vi "ULx Create Channel (AI-Temperature).vi"(0 "task in":refnum<k24>, 5 "physical channels":refnum<k21>, 7 "units":i32(ring) items=["degC", "degF", "kelvin", "raw"], 11 "error in":errorcluster) -> (4 "task out":refnum<k24>, 15 "error out":errorcluster)   [LabVIEW 2020]
doc: "Creates channel(s) to measure temperature."
uses:
  C:/Users/William/Documents/LV 2020 builds/LeaktestDAQ/Source-v33/ULx_LV.dll
  ULx_LV.dll
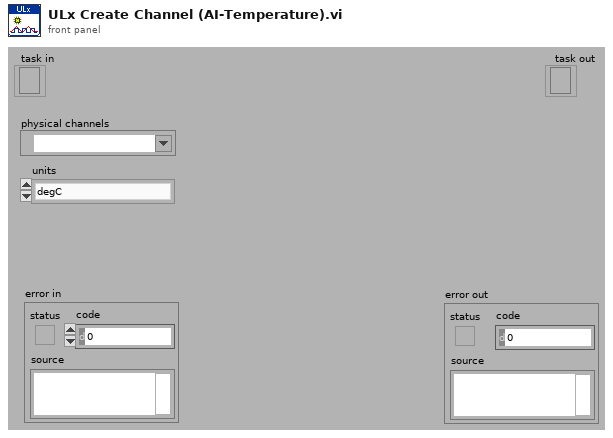
[diagram p1: front panel]
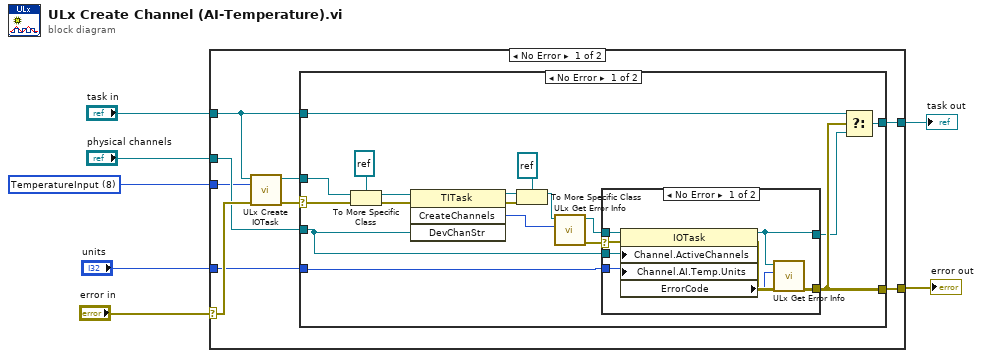
[diagram p0: block diagram]
diagram:
  w2 = 8 items=["AnalogInput", "AnalogOutput", "DigitalInput", "DigitalOutput", "CounterInput", "CounterOutput", "CompositeInput", "CompositeOutput", "TemperatureInput"] ("taskType")
  n1 = case shown="No Error" "error in" {
    selector: "error in" -> [w16 w47]
    tunnel: "task in" -> [w8 w46]
    tunnel: "physical channels" -> [w11 _]
    tunnel: [w14 w46] -> w5
    tunnel: [w13 w47] -> w4
    tunnel: w2 -> [w10 _]
    tunnel: "units" -> [w9 _]
    frame No Error {
      n2 = call "ULx Create IOTask.vi"("error in"=w16, "taskType"=w10, "i/o task in"=w8) -> ("error out"=w15:errorcluster, "i/o task out"=w12:refnum<k24>)  [unwired: 7 in]
      n3 = case shown="No Error" w15 {
        selector: w15 -> [w31 w45]
        tunnel: [w18 w45] -> w13
        tunnel: [w20 w44] -> w14
        tunnel: w12 -> [w29 _]
        tunnel: w11 -> [w25 _]
        tunnel: w9 -> [w26 _]
        tunnel: w8 -> [w19 w44]
        frame No Error {
          n4 = To More Specific Class(target class=refnum<k24> refnum, reference=w29, error in=w31) -> (specific class reference=w32:refnum<k24>, error out=w30:errorcluster)
          n5 = invoke class="TITask" method="CreateChannels"(reference=w32, error in=w30, "DevChanStr"=w25) -> (reference out=w23:refnum<k24>, error out=w22:errorcluster, "CreateChannels"=w28:i32)  [unwired: 1 in, 1 out]
          n6 = To More Specific Class(target class=refnum<k24> refnum, reference=w23, error in=w22) -> (specific class reference=w21:refnum<k24>)  [unwired: 1 out]
          n7 = call "ULx Get Error Info.vi"("ErrorCode"=w28, "task in"=w21) -> ("error out"=w27:errorcluster)  [unwired: 9 in]
          n8 = case shown="No Error" w27 {
            selector: w27 -> [w41 w43]
            tunnel: w21 -> [w40 w42]
            tunnel: w26 -> [w35 _]
            tunnel: w25 -> [w39 _]
            tunnel: [w36 w43] -> w18
            tunnel: [w34 w42] -> w17
            frame No Error {
              n9 = property class="IOTask"(reference=w40, error in=w41, "Channel.ActiveChannels"=w39, "Channel.AI.Temp.Units"=w35) -> (reference out=w34:refnum<k24>, error out=w37:errorcluster, "ErrorCode"=w38:i32)
              n10 = call "ULx Get Error Info.vi"("error in"=w37, "ErrorCode"=w38, "task in"=w34) -> ("error out"=w36:errorcluster)  [unwired: 8 in]
            }
            frame Error {
            }
          }
          n11 = Select(t=w19, s=w18, f=w17) -> (s? t:f=w20:refnum<k24>)
        }
        frame Error {
        }
      }
    }
    frame Error {
    }
  }
  "error out" <- w4
  "task out" <- w5
